vi "Get Rects.vi"(8 "error in (no error)":errorcluster, 11 "ParseSVG in":refnum<class "ParseSVG.lvclass">) -> (0 "error out":errorcluster, 3 "ParseSVG out":refnum<class "ParseSVG.lvclass">)   [LabVIEW 2019, in "ParseSVG.lvclass"]
uses:
  ParseSVG.lvclass
  Rect.ctl
  ParseSVG.lvclass/ParseSVG.ctl
  Read RawXML.vi
  <userlib>/_OpenG.lib/lvdata/lvdata.llb/Get Data Name__ogtk.vi
  <userlib>/_OpenG.lib/lvdata/lvdata.llb/Get Cluster Element Names__ogtk.vi
  <userlib>/_OpenG.lib/lvdata/lvdata.llb/Array of VData to VCluster__ogtk.vi
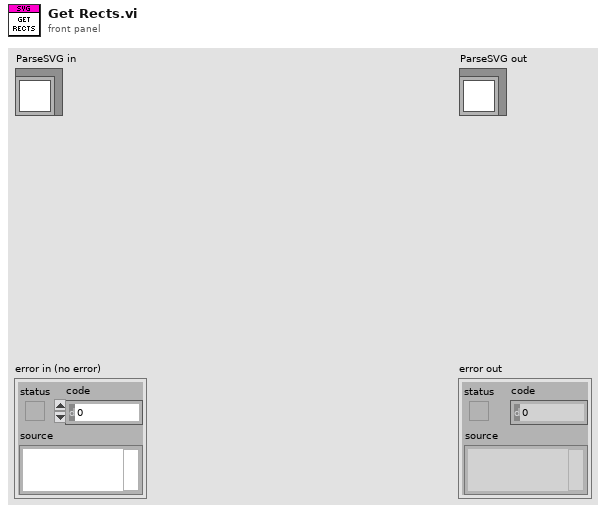
[diagram p1: front panel]
types:
  T1 = typedef "ParseSVG.lvclass/Rect.ctl" = cluster{"style":string, "transform":string, "x":string, "y":string, "width":string, "height":string, "rx":string, "ry":string, "id":string}
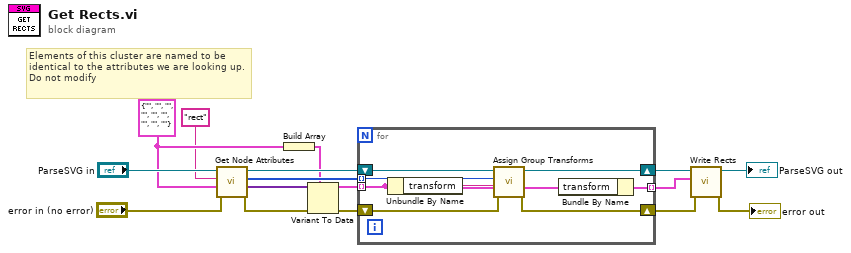
[diagram p0: block diagram]
diagram:
  w11 = T1 {"style"="", "transform"="", "x"="", "y"="", "width"="", "height"="", "rx"="", "ry"="", "id"=""} ("Rect")
  # "Elements of this cluster are named to be identical to the attributes we are looking up. Do not modify"
  n1 = call "Get Node Attributes.vi"("error in (no error)"="error in (no error)", "Attributes Cluster"=w11, "Node Name (exact)"="rect", "ParseSVG in"="ParseSVG in") -> ("error out"=w9:errorcluster, "[Attributes Cluster]"=w12:variant[], "Positions"=w7:i32[], "ParseSVG out"=w8:refnum<class "ParseSVG.lvclass">)  [unwired: 4 in]
  n2 = Build Array(w11) -> (w1:T1[])
  n3 = Variant To Data(error in=w9, type=w1, Variant=w12) -> (data=w6:T1[], error out=w5:errorcluster)
  n4 = for {
    shift-right: [w24] -> w3
    shift-left: w8 -> [w25]
    shift-right: [w22] -> w4
    shift-left: w5 -> [w23]
    tunnel: w6 -> [w19] mode=indexing
    tunnel: w7 -> [w20] mode=indexing
    tunnel: [w17] -> w2 mode=indexing
    n5 = Unbundle By Name(w19) -> ("transform"=w21:string)
    n6 = call "Assign Group Transforms.vi"("error in (no error)"=w23, "transform in"=w21, "position"=w20, "ParseSVG in"=w25) -> ("error out"=w22:errorcluster, "transform out"=w18:string, "ParseSVG out"=w24:refnum<class "ParseSVG.lvclass">)  [unwired: 5 in]
    n7 = Bundle By Name(cluster=w19, "transform"=w18) -> (w17:T1)
  }
  n8 = call "Write Rects.vi"("error in (no error)"=w4, "Rects"=w2, "ParseSVG in"=w3) -> ("error out"=→"error out":errorcluster, "ParseSVG out"=→"ParseSVG out":refnum<class "ParseSVG.lvclass">)  [unwired: 7 in]
